vi "Get DBAlias.vi"(8 "error in (no error)":errorcluster, 10 "DB Alias":string, 11 "Device Item Ref in":T1 format="%.0x") -> (0 "error out":errorcluster, 2 "Alias":string, 3 "Device Item Ref out":T1 format="%.0x")   [LabVIEW 2018, in "CAN Gateway System Explorer.lvlib"]
uses:
  CAN Gateway System Explorer.lvlib
  <vilib>/NI Veristand/Custom Device API/Custom Device Item Ref.ctl
  Shared/Constants.vi
  <vilib>/NI Veristand/Custom Device Tools/Custom Device Utility Library/NI VeriStand - Search for Item by GUID.vi
  <vilib>/NI Veristand/Custom Device Tools/Custom Device Utility Library/NI VeriStand - Search for Item by Name.vi
  <vilib>/NI/NI VeriStand Advanced SysDef API/_SubVIs/SysDef.Property.Get.String.vi
  <vilib>/NI Veristand/Custom Device Tools/Custom Device Utility Library/Custom Device Utility Library.lvlib
  Shared/CAN Gateway Shared.lvlib
  <vilib>/NI/NI VeriStand Advanced SysDef API/SysDef API/Advanced System Definition.lvlib
  <vilib>/NI Veristand/Custom Device API/Custom Device API.lvlib
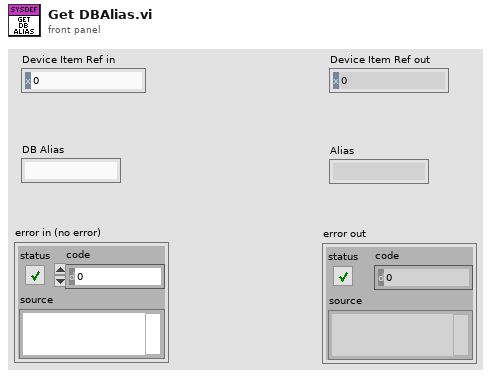
[diagram p1: front panel]
types:
  T1 = typedef "Custom Device API.lvlib/Custom Device Item Ref.ctl" = u64
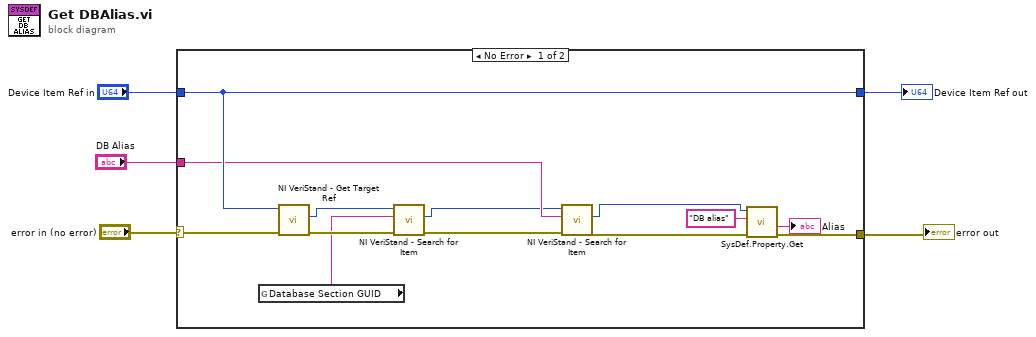
[diagram p0: block diagram]
diagram:
  n1 = case shown="No Error" "error in (no error)" {
    selector: "error in (no error)" -> [w18 w20]
    tunnel: "Device Item Ref in" -> [w8 w19]
    tunnel: [w8 w19] -> w3
    tunnel: [w13 w20] -> w2
    tunnel: "DB Alias" -> [w7 _]
    frame No Error {
      n2 = global read "Constants.vi" "Database Section GUID"() -> (w16:string)
      n3 = call <vilib>:"NI VeriStand - Get Target Ref.vi"("error in"=w18, "Item Ref in"=w8) -> ("error out"=w17:errorcluster, "Target Ref"=w15:T1)  [unwired: 6 in, 2 out]
      n4 = call-poly <vilib>:"NI VeriStand - Search for Item.vi"("error in"=w17, "Item GUID"=w16, "Section Ref in"=w15) -> ("error out"=w11:errorcluster, "Item Ref"=w6:T1)  [unwired: 5 in, 2 out]
      n5 = call-poly <vilib>:"NI VeriStand - Search for Item.vi"("error in"=w11, "Item Name"=w7, "Section Ref in"=w6) -> ("error out"=w9:errorcluster, "Item Ref"=w10:T1)  [unwired: 5 in, 2 out]
      n6 = call-poly <vilib>:"SysDef.Property.Get.vi"("error in (no error)"=w9, "Property Name"="DB alias", "nodeID"=w10) -> ("error out"=w13:errorcluster, "Value out"=→"Alias":string)  [unwired: 5 in, 2 out]
    }
    frame Error {
    }
  }
  "error out" <- w2
  "Device Item Ref out" <- w3
